vi "Read TDMS_Report.vi"   [LabVIEW 2009]
doc: "This allows the user to easily view a TDMS report that is created.\n\nAAL 9/09"
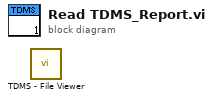
[diagram p0: block diagram]
diagram:
  n1 = call <vilib>:"TDMS - File Viewer.vi"() -> ()  [unwired: 2 in, 6 out]
